vi "editDialog.vi"(0 "reference":refnum<class "UseCaseNode.lvclass">, 1 "insidePackageNode":bool, 5 "error in (no error)":errorcluster) -> (14 "reference out":refnum<class "UseCaseNode.lvclass">, 15 "changeConnection":T1, 16 "cancel":bool, 19 "error out":errorcluster)   [LabVIEW 2020, in "UseCaseNode.lvclass"]
doc: "Edit Dialog"
uses:
  <resource>/Framework/Providers/Open_GDS/UML/UseCaseNode_class/UseCaseNode.lvclass
  C:/Program Files (x86)/National Instruments/LabVIEW 2020/resource/Framework/Providers/Open_GDS/UML/AbstractNode_class/AbstractNode.lvclass
  <resource>/Framework/Providers/Open_GDS/UML/AbstractNode_class/private/NodeConnectionStatsType.ctl
  <resource>/Framework/Providers/Open_GDS/UML/ContextHelp/ContextHelp_HelpTexts.ctl
  <resource>/Framework/Providers/Open_GDS/UML/MultiLineString_class/MultiLineString.lvclass
  <resource>/Framework/Providers/Open_GDS/UML/AbstractNode_class/AbstractNode.lvclass
panel:
  in  "OK Button":bool
  in  "Cancel Button":bool
  in  "Help":bool
  in  "connection":bool caption="Connect to System"
  in  "Use Case text":string
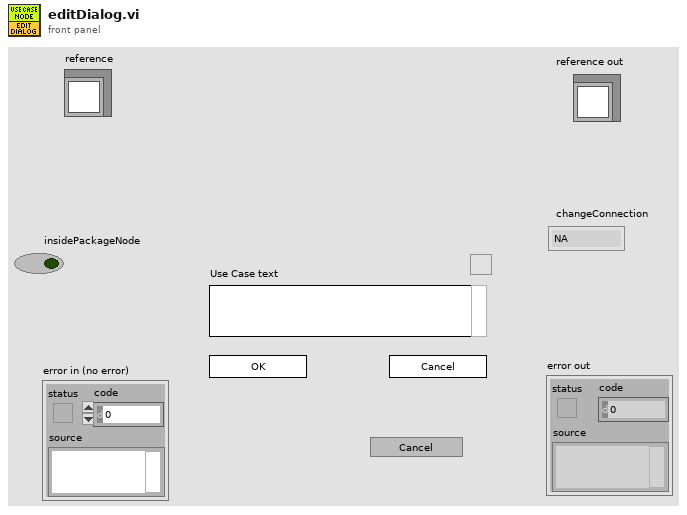
[diagram p1: front panel]
types:
  T1 = typedef "AbstractNode.lvclass/NodeConnectionStatsType.ctl" = enum16{"NA", "Connect", "DisConnect"}
  T2 = typedef "ContextHelp_HelpTexts.ctl" = enum16{"None(Hide)", "Default", "Help", "Welcome", "GettingStarted", "ClassDiagram_Help", "SequenceDiagram_Help", "UseCaseDiagram_Help", "BSelect", "BClass", "BInterface", "BPackage", "BNote", "BDependency", "BInheritance", "BInterfaceImplementation", "BAssociation", "BAggregation", "BCompAggregation", "BNoteConnector", "BObject", "BActionBar", "BCall", "BSystem", "BActor", "BUseCase", "BGeneralization", "BIncludes", "BExtends", "BUseCaseDiagramAssociation", "ClassRelationshipEdge editDialog_Bent Style", "ClassRelationshipEdge editDialog_RelationType", "ClassRelationshipEdge editDialog_Reverse association", "ClassRelationshipEdge editDialog_Start label", "ClassRelationshipEdge editDialog_Middle label", "ClassRelationshipEdge editDialog_End label", "UMLEditor reversedEngineering_Pathes", "ReversedEngineering StateReverseDialog_Help", "ReversedEngineering StateQueuedSettings_Help", "UMLEditor reversedEngineering_AddTopVIs", "UMLEditor reversedEngineering_AddClasses", "UMLEditor reversedEngineering_AddDirs", "UMLEditor reversedEngineering_Recursively", "UMLEditor reversedEngineering_Remove", "UMLEditor reversedEngineering_ClearList", "UMLEditor reversedEngineering_HideSubAss", "UMLEditor reversedEngineering_CreateTypes", "UMLEditor reversedEngineering_OnlyInheritance", "UMLEditor reversedEngineering_CreateApplication", "UMLEditor reversedEngineering_OK", "UMLEditor reversedEngineering_Cancel", "UMLEditor reversedEngineering_Help", "UMLEditor createWizardScriptFile_ScriptfilePath", "UMLEditor createWizardScriptFile_ClassPath", "UMLEditor createWizardScriptFile_Use", "UMLEditor createWizardScriptFile_PrivateDirName", "UMLEditor createWizardScriptFile_DirAppend", "UMLEditor createWizardScriptFile_Separator Character", "UMLEditor createWizardScriptFile_OK", "UMLEditor createWizardScriptFile_Cancel", "UMLEditor createWizardScriptFile_Help", "ClassNode editDialog_Class Name", "InterfaceNode editDialog_Class Name", "ClassNode editDialog_Attribute", "ClassNode editDialog_Methods", "InterfaceNode editDialog_Methods", "ClassNode editDialog_connection", "InterfaceNode editDialog_connection", "ClassNode editDialog_StereoType", "ClassNode editDialog_ShowAttrib", "ClassNode editDialog_ShowMethods", "ClassNode editDialog_ClassPath", "ClassNode editDialog_AddAttribute", "ClassNode editDialog_AddMethod", "InterfaceNode editDialog_AddMethod", "ClassNode AttributeGuide_AttributeName", "ClassNode AttributeGuide_Array?", "ClassNode AttributeGuide_Data Type", "ClassNode AttributeGuide_RefName", "ClassNode AttributeGuide_Preview", "ClassNode AttributeGuide_OK", "ClassNode AttributeGuide_Cancel", "ClassNode MethodGuide_Visibility", "ClassNode MethodGuide_Method Name", "ClassNode MethodGuide_Preview", "ClassNode MethodGuide_OK", "ClassNode MethodGuide_Cancel", "CallNode EditCallProperties_AllButtons", "ObjectNode EditObjectlProperties_AllButtons", "ActorNode EditActorProperties_AllButtons", "UseCaseRelationshipNode EditUseCaselProperties_AllButtons", "UseCaseNode EditUseCaselProperties_AllButtons", "SystemNode EditSystemProperties_AllButtons", "ReversedEngineering UpdateAttributes_AllButtons", "StateNode editDialog_AllButtons", "StateTransition editDialog_AllButtons", "ArrangeNodes Main_Picture", "ArrangeNodes Main_Zoom", "ArrangeNodes Main_Auto Zoom", "ArrangeNodes Main_shorten", "ArrangeNodes Main_Min Length", "ArrangeNodes Main_Max Length", "ArrangeNodes Main_increase", "ArrangeNodes Main_decrease", "ArrangeNodes Main_Shake", "ArrangeNodes Main", "BState", "BInitialState", "BFinalState", "BStateTransition", "StateDiagram_Help", "StateDiagram_PropertiesAllButtons", "ReversedEngineering StateReverseDialog_ClearStates", "ReversedEngineering StateReverseDialog_UseQueuedStateMachines", "ReversedEngineering StateReverseDialog_QueuedSettings", "ReversedEngineering StateReverseDialog_SearchForVIs", "ReversedEngineering StateReverseDialog_SearchCriteria", "OptionsDialog_ClassBasePath", "OptionsDialog_VIPath", "OptionsDialog_ApplicationPath", "OptionsDialog_WizDir", "OptionsDialog_IniFilePath", "OptionsDialog_DefineColors", "OptionsDialog_Help", "OptionsDialog_CreateTypes", "ClassRelationshipEdge editDialog_SplitWire"}
  T3 = typedef "UseCaseNode.lvclass/ObjectAttributes.ctl" = cluster{"name":refnum<class "MultiLineString.lvclass">, "DEFAULT_WIDTH":i32, "DEFAULT_HEIGHT":i32}
  T4 = typedef "AbstractNode.lvclass/ObjectAttributes.ctl" = cluster{"parent":refnum<class "AbstractNode.lvclass">, "children":refnum<class "AbstractNode.lvclass">[], "Hidden":bool}
  T5 = typedef "ContextHelp_ShowType.ctl" = cluster{"Header":string, "Picture":picture, "Text":string}
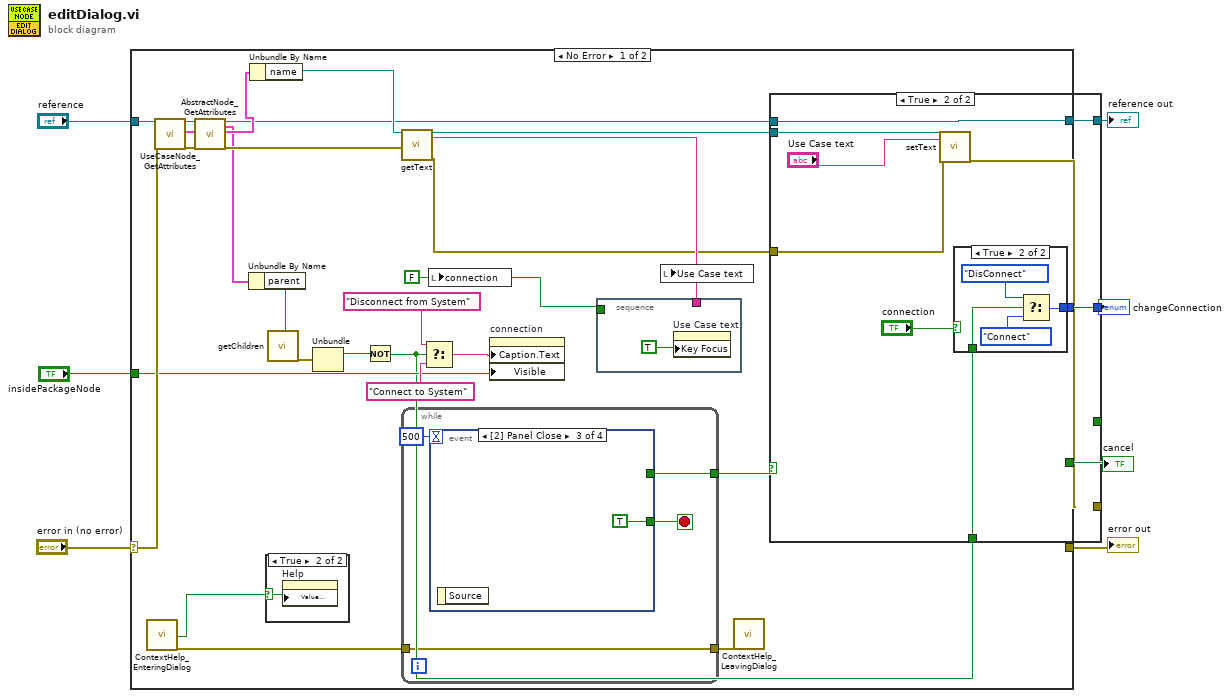
[diagram p0: block diagram]
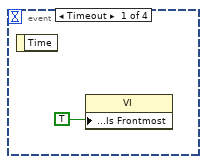
[diagram p3: hidden frame]
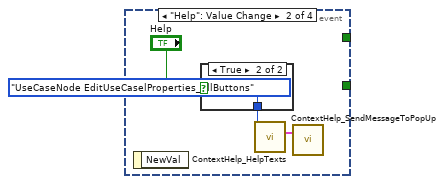
[diagram p4: hidden frame]
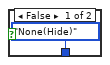
[diagram p5: hidden frame]
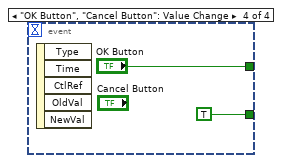
[diagram p6: hidden frame]
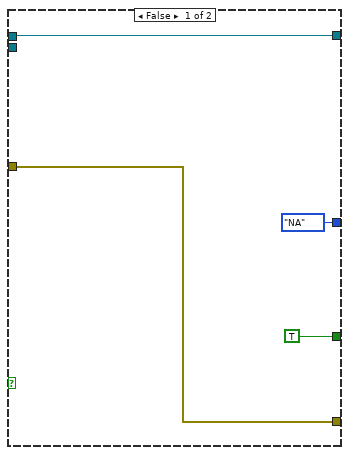
[diagram p7: hidden frame]
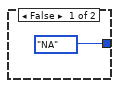
[diagram p8: hidden frame]
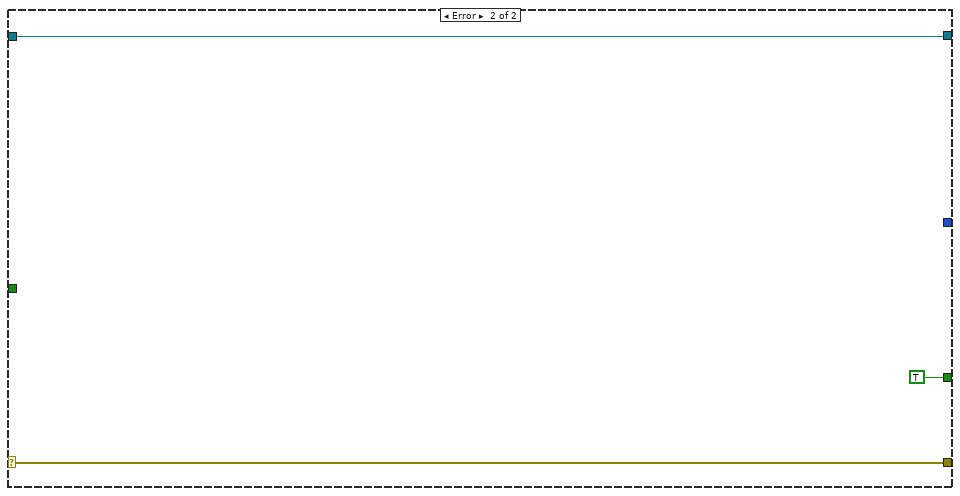
[diagram p9: hidden frame]
diagram:
  n1 = case shown="No Error" "error in (no error)" {
    selector: "error in (no error)" -> [w33 w70]
    tunnel: "reference" -> [w34 w71]
    tunnel: [w36 w70] -> w5
    tunnel: [w35 w71] -> w4
    tunnel: [w29 _] -> w3
    tunnel: "insidePackageNode" -> [w25 _]
    tunnel: [w23 TRUE ("Key Focus")] -> w1
    frame No Error {
      w24 = FALSE ("connection")
      n2 = call <resource>:"ContextHelp_EnteringDialog.vi"() -> ("HelpStatus"=w18:bool, "error out"=w20:errorcluster)  [unwired: 3 in, 15 out]
      n3 = call <resource>:"UseCaseNode_GetAttributes.vi"("reference in"=w34, "error in (no error)"=w33) -> ("reference out"=w12:refnum<class "UseCaseNode.lvclass">, "Data"=w13:T3, "error out"=w11:errorcluster)  [unwired: 1 in, 14 out]
      n4 = call <resource>:"AbstractNode_GetAttributes.vi"("reference in"=w12, "error in (no error)"=w11) -> ("reference out"=w9:refnum<class "UseCaseNode.lvclass">, "Data"=w8:T4, "error out"=w10:errorcluster)  [unwired: 14 in, 1 out]
      n5 = Unbundle By Name(w8) -> ("parent"=w17:refnum<class "AbstractNode.lvclass">)
      n6 = Unbundle By Name(w13) -> ("name"=w30:refnum<class "MultiLineString.lvclass">)
      n7 = case shown="True" w18 {
        selector: w18 -> [_ w37]
        frame False {
        }
        frame True {
          n8 = property on="Help" class="Bool (strict)"("Value (Signaling)"=w37) -> ()  [unwired: 2 in, 2 out]
        }
      }
      n9 = call-dynamic "getChildren.vi"("reference"=w17) -> ("error out"=w16:errorcluster)  [unwired: 15 in, 3 out]
      n10 = Unbundle(w16) -> ("status"=w15:bool)  [unwired: 2 out]
      n11 = Not(x=w15) -> (.not. x?=w14:bool)
      n12 = call-dynamic "getText.vi"("reference"=w30, "error in (no error)"=w10) -> ("reference out"=w32:refnum<class "MultiLineString.lvclass">, "text"=w31:string, "error out"=w22:errorcluster)  [unwired: 15 in]
      n13 = while {
        tunnel: [w41] -> w19
        tunnel: [w39] -> w21
        tunnel: w20 -> [w39]
        stop <- w40 stop-if-true
        n14 = event shown="[2] Panel Close" {
          selector: _ -> [_ _ _ _]
          dyn-events: _ -> [_ _ _ _]
          timeout: 500 -> [_ _ _ _]
          tunnel: [_ _ _ "OK Button"] -> w41
          tunnel: [_ _ TRUE TRUE] -> w40
          event Timeout {
            n15 = event-data() -> ()  [unwired: 2 out]
            n16 = property class="VI"("Front Panel Window:Is Frontmost"=TRUE) -> ()  [unwired: 2 in, 2 out]
          }
          event "Help": Value Change {
            n17 = event-data() -> ()  [unwired: 2 out]
            n18 = case shown="True" "Help" {
              tunnel: [ContextHelp_HelpTexts."None(Hide)" ("HelpText") ContextHelp_HelpTexts."UseCaseNode EditUseCaselProperties_AllButtons" ("HelpText")] -> w44
              frame False {
              }
              frame True {
              }
            }
            n19 = call <resource>:"ContextHelp_HelpTexts.vi"("HelpText (enum or string)"=w44) -> ("HelpOut"=w45:T5)  [unwired: 18 out]
            n20 = call <resource>:"ContextHelp_SendMessageToPopUp.vi"("PopUpMessage"=w45) -> ()  [unwired: 2 in, 17 out]
          }
          event Panel Close {
            n21 = event-data() -> ()  [unwired: 2 out]
          }
          event "OK Button", "Cancel Button": Value Change {
            n22 = event-data() -> ()  [unwired: 6 out]
          }
        }
      }
      n23 = Select(t="Disconnect from System", s=w14, f="Connect to System") -> (s? t:f=w28:string)
      n24 = local write "connection"(w24) -> ()
      n25 = property on="connection" class="Bool (strict)"("Caption.Text"=w28, "Visible"=w25) -> ()  [unwired: 2 in, 2 out]
      n26 = stacked-sequence {
        tunnel: w31 -> [_]
        tunnel: w24 -> [_]
        frame #0 {
          n27 = property on="Use Case text" class="Str"("Key Focus"=TRUE) -> ()  [unwired: 2 in, 2 out]
        }
      }
      n28 = local write "Use Case text"(w31) -> ()
      n29 = call <resource>:"ContextHelp_LeavingDialog.vi"("error in (no error)"=w21) -> ()  [unwired: 2 in, 17 out]
      n30 = case shown="True" w19 {
        tunnel: [w53 w59] -> w36
        tunnel: [w54 w60] -> w35
        tunnel: w9 -> [w54 w60]
        tunnel: w32 -> [_ w62]
        tunnel: w22 -> [w53 w55]
        tunnel: [enum16{"NA", "Connect", "DisConnect"}."NA" ("changeConnection") w57] -> w29
        tunnel: w14 -> [_ w56]
        tunnel: [TRUE ("Key Focus") _] -> w23
        frame False {
        }
        frame True {
          n31 = call-dynamic "setText.vi"("reference"=w62, "text"="Use Case text", "error in (no error)"=w55) -> ("error out"=w59:errorcluster)  [unwired: 15 in, 1 out]
          n32 = case shown="True" "connection" {
            tunnel: [enum16{"NA", "Connect", "DisConnect"}."NA" ("changeConnection") w66] -> w57
            tunnel: w56 -> [_ w67]
            frame False {
            }
            frame True {
              n33 = Select(t=enum16{"NA", "Connect", "DisConnect"}."DisConnect" ("changeConnection"), s=w67, f=enum16{"NA", "Connect", "DisConnect"}."Connect" ("changeConnection")) -> (s? t:f=w66:enum16{"NA", "Connect", "DisConnect"})
            }
          }
        }
      }
    }
    frame Error {
    }
  }
  "reference out" <- w4
  "error out" <- w5
  "changeConnection" <- w3
  "cancel" <- w1
